vi "IsBlank.vi"(1 "Column":i32, 2 "Row":i32, 3 "Board":i32[][](array[numeric])) -> (0 "Boolean":bool)   [LabVIEW 2014]
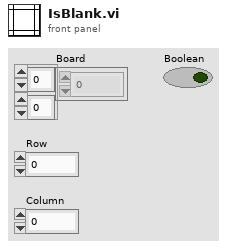
[diagram p1: front panel]
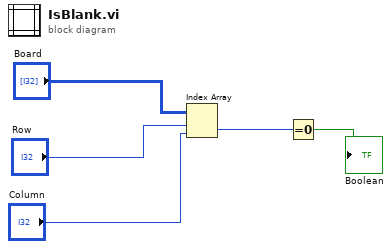
[diagram p0: block diagram]
diagram:
  n1 = Index Array(array="Board", index (row)="Row", index (col)="Column") -> (element=w4:i32)
  n2 = Equal To 0?(x=w4) -> (x = 0?=→"Boolean":bool)
